vi "Cache Data Point.vi"(0 "Reset?":bool, 1 "Pass?":bool, 3 "Current Cache":T1[](array[typedef]), 4 "New Cache":T1, 5 "Channels Size":i32, 6 "Channel Index":i32, 7 "error in (no error)":errorcluster) -> (20 "Cache out":T1[](array[typedef]), 27 "error out":errorcluster)   [LabVIEW 2026, in "Processing_Engine.lvlib"]
doc: "Overwrite current failed data point with new failed data point into cache."
uses:
  Processing_Engine.lvlib
  controls/Messaging Payloads/Processed Calibration Point.ctl
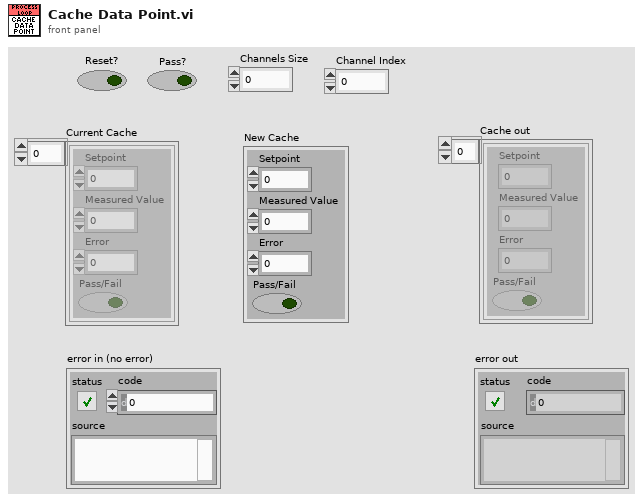
[diagram p1: front panel]
types:
  T1 = typedef "Processed Calibration Point.ctl" = cluster{"Setpoint":dbl, "Measured Value":dbl, "Error":dbl, "Pass/Fail":bool}
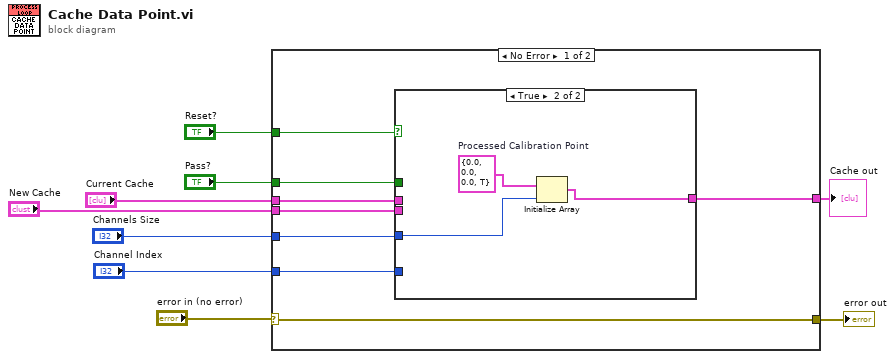
[diagram p0: block diagram]
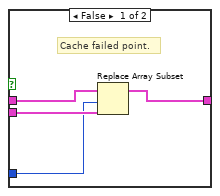
[diagram p3: hidden frame]
diagram:
  n1 = case shown="No Error" "error in (no error)" {
    selector: "error in (no error)" -> [w13 w32]
    tunnel: "Current Cache" -> [w17 w31]
    tunnel: [w16 w31] -> w2
    tunnel: "New Cache" -> [w15 _]
    tunnel: "Pass?" -> [w14 _]
    tunnel: [w13 w32] -> w5
    tunnel: "Reset?" -> [w12 _]
    tunnel: "Channels Size" -> [w11 _]
    tunnel: "Channel Index" -> [w10 _]
    frame No Error {
      n2 = case shown="True" w12 {
        tunnel: w17 -> [w22 _]
        tunnel: [w21 w28] -> w16
        tunnel: w15 -> [w20 _]
        tunnel: w14 -> [w19 _]
        tunnel: w11 -> [_ w30]
        tunnel: w10 -> [w18 _]
        frame False {
          n3 = case shown="True" w19 {
            tunnel: w20 -> [w26 _]
            tunnel: [w24 w27] -> w21
            tunnel: w22 -> [w25 w27]
            tunnel: w18 -> [w23 _]
            frame False {
              # "Cache failed point."
              n4 = Replace Array Subset(array=w25, new element=w26, index=w23) -> (w24:T1[])
            }
            frame True {
              # "Maintain failed cache."
            }
          }
        }
        frame True {
          w29 = T1 {"Setpoint"=0.0, "Measured Value"=0.0, "Error"=0.0, "Pass/Fail"=TRUE}  # Processed Calibration Point
          n5 = Initialize Array(w29, w30) -> (w28:T1[])
        }
      }
    }
    frame Error {
    }
  }
  "error out" <- w5
  "Cache out" <- w2
